vi "Teleop.vi"(10 "Match Info":T1={"Autonomous Elapsed Seconds"=0.0, "TeleOp Elapsed Seconds"=0.0, "Disabled Elapsed Seconds"=0.0, "Visited Autonomous"=FALSE, "Visited TeleOp"=FALSE, "Visited Disabled"=FALSE, "Autonomous Settings"={"Autonomous Style"=enum."Independent", "VI Refnum"=refnum}}, 11 "Call Context":T2) -> ()   [LabVIEW 2019]
doc: "This VI is called for each TeleOp packet received from the DS where the robot is not disabled. It is often used to read from the joysticks and update I/O or to update setpoints for timed control loops. It should complete and return within 20 milliseconds or it may miss DS packets."
uses:
  <vilib>/Rock Robotics/WPI/DriverStation/WPI_DriverStationDerivedRobotMode.ctl
  <vilib>/Rock Robotics/WPI/DriverStation/WPI_DriverStationMatch Info.ctl
  Robot Global Data.vi
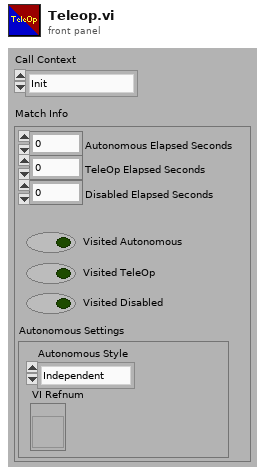
[diagram p1: front panel]
types:
  T1 = typedef "WPI_DriverStationMatch Info.ctl" = cluster{"Autonomous Elapsed Seconds":dbl, "TeleOp Elapsed Seconds":dbl, "Disabled Elapsed Seconds":dbl, "Visited Autonomous":bool, "Visited TeleOp":bool, "Visited Disabled":bool, "Autonomous Settings":cluster{"Autonomous Style":enum16{"Iterative", "Independent"}, "VI Refnum":refnum<vi>}}
  T2 = typedef "WPI_DriverStationDerivedRobotMode.ctl" = enum16{"Init", "Execute", "Stop"}
  T3 = typedef "WPI_JoystickDevRef.ctl" = cluster{"Device":T4}
  T4 = typedef "WPI_JoystickDeviceEnum.ctl" = enum16{"USB 0", "USB 1", "USB 2", "USB 3", "USB 4", "USB 5"}
  T5 = typedef "Color Sensor V3 DevRef.ctl" = cluster{"I2CDevRef":T6}
  T6 = typedef "WPI_I2CDevRef.ctl" = cluster{"DevStatus":errorcluster, "Device Address":u8, "Handle":i32, "I2C Bus":T7}
  T7 = typedef "i2c_bus.ctl" = enum16{"I2C On-Board", "I2C MXP", "Invalid"}
  T8 = typedef "WPI_EncoderDevRef.ctl" = cluster{"DevStatus":errorcluster, "EncoderIndex":T9, "CounterIndex":T10, "DistancePerCount":dbl, "Decoding Type":T11}
  T9 = typedef "FPGA_EncoderIdx.ctl" = enum8{"Enc 0", "Enc 1", "Enc 2", "Enc 3", "Enc 4", "Enc 5", "Enc 6", "Enc 7", "Invalid"}
  T10 = typedef "FPGA_CounterCtrSystemIndex.ctl" = enum8{"Ctr 0", "Ctr 1", "Ctr 2", "Ctr 3", "Ctr 4", "Ctr 5", "Ctr 6", "Ctr 7", "Invalid"}
  T11 = typedef "WPI_EncoderType.ctl" = enum16{"1x", "2x", "4x"}
  T12 = typedef "WPI_MotorControlDeviceRef.ctl" = cluster{"DeviceStatus":errorcluster, "Type":T13, "PWM":cluster{"PWM Channel":T14, "DeadBand":T15}, "CAN":cluster{"Device Number":u8, "SetOutput VI Ref":variant, "GetOutput VI Ref":variant, "Enable VI Ref":variant, "Disable VI Ref":variant, "Data":variant}, "Invert":bool, "DIO PWM":cluster{"PWM \"Enable\" Channel":T14, "DIOChannel":T16, "PWM Rate":dbl}}
  T13 = typedef "WPI_MotorControlType.ctl" = enum16{"PWM", "CAN", "DIO PWM"}
  T14 = typedef "FPGA_DIOPWMChannel.ctl" = enum8{"PWM 0", "PWM 1", "PWM 2", "PWM 3", "PWM 4", "PWM 5", "PWM 6", "PWM 7", "PWM 8", "PWM 9", "PWM MXP 0", "PWM MXP 1", "PWM MXP 2", "PWM MXP 3", "PWM MXP 4", "PWM MXP 5", "PWM MXP 6", "PWM MXP 7", "PWM MXP 8", "PWM MXP 9", "Invalid"}
  T15 = typedef "WPI_PWMDeadband.ctl" = cluster{"Name":string, "maxPositivePwm":i32, "minPositivePwm":i32, "centerPwm":i32, "maxNegativePwm":i32, "minNegativePwm":i32, "angularRange":u16}
  T16 = typedef "FPGA_DIOChannel.ctl" = enum8{"DIO 0", "DIO 1", "DIO 2", "DIO 3", "DIO 4", "DIO 5", "DIO 6", "DIO 7", "DIO 8", "DIO 9", "DIO MXP 0", "DIO MXP 1", "DIO MXP 2", "DIO MXP 3", "DIO MXP 4", "DIO MXP 5", "DIO MXP 6", "DIO MXP 7", "DIO MXP 8", "DIO MXP 9", "DIO MXP 10", "DIO MXP 11", "DIO MXP 12", "DIO MXP 13", "DIO MXP 14", "DIO MXP 15", "SPI Port CS1", "SPI Port CS2", "SPI Port CS3", "SPI Port MISO", "SPI Port MOSI", "Invalid"}
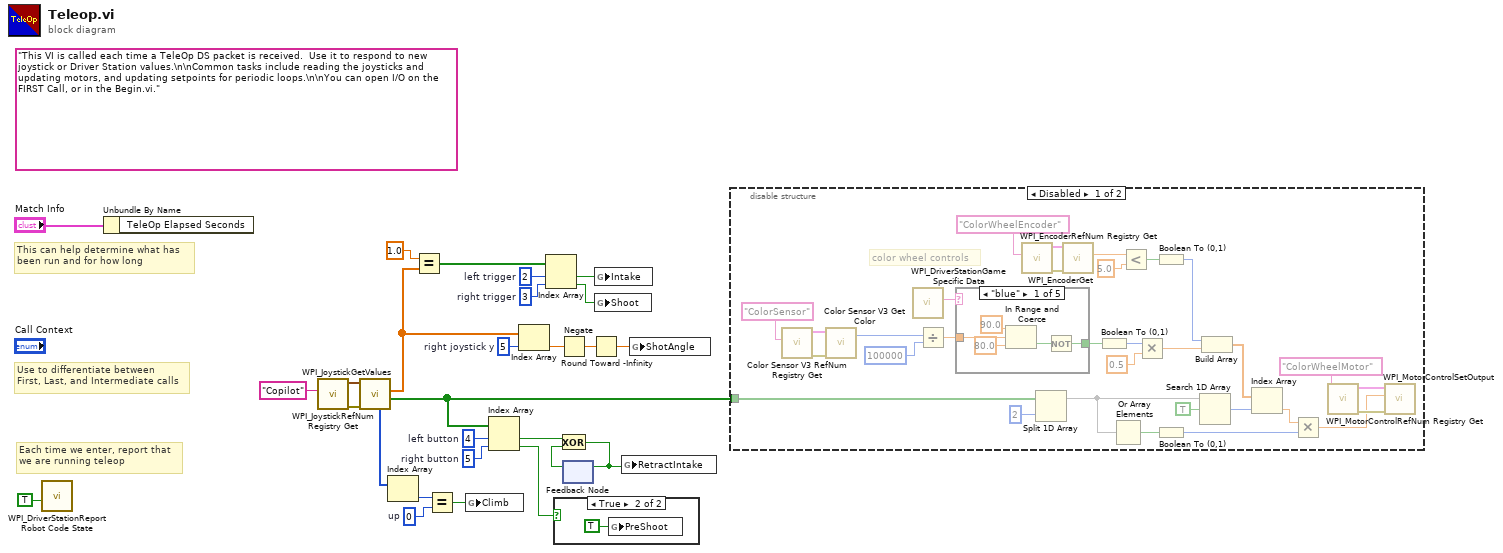
[diagram p0: block diagram]
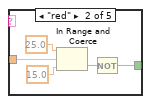
[diagram p3: hidden frame]
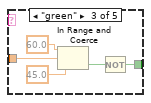
[diagram p4: hidden frame]
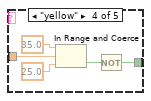
[diagram p5: hidden frame]
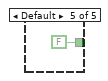
[diagram p6: hidden frame]
diagram:
  w11 = 5  # right joystick y
  w16 = i16 0  # up
  w22 = 5  # right button
  w23 = 4  # left button
  w24 = 3  # right trigger
  w25 = 2  # left trigger
  (unwired) "This VI is called each time a TeleOp DS packet is received.  Use it to respond to new joystick or Driver Station values.\n\nCommon tasks include reading the joysticks and updating motors, and updating setpoints for periodic loops.\n\nYou can open I/O on the FIRST Call, or in the Begin.vi."
  # "Each time we enter, report that\nwe are running teleop"
  # "Use to differentiate between\nFirst, Last, and Intermediate calls"
  # "This can help determine what has\nbeen run and for how long"
  n1 = call <vilib>:"WPI_DriverStationReport Robot Code State.vi"("TeleOp"=TRUE ("Autonomous")) -> ()  [unwired: 10 in, 1 out]
  n2 = Unbundle By Name("Match Info") -> ()  [unwired: 1 out]
  n3 = call <vilib>:"WPI_JoystickRefNum Registry Get.vi"("refnum name"="Copilot") -> ("error out"=w1:errorcluster, "JoystickDevRef"=w2:T3)  [unwired: 9 in]
  n4 = call <vilib>:"WPI_JoystickGetValues.vi"("error in (no error)"=w1, "JoystickDevRef"=w2) -> ("Buttons"=w13:bool[], "Axes"=w10:dbl[], "POVs"=w18:i16[])  [unwired: 5 in, 2 out]
  n5 = Index Array(array=w18) -> (element=w17:i16)  [unwired: 1 in]
  n6 = Equal?(x=1.0, y=w10) -> (x = y?=w21:bool[])
  n7 = Equal?(x=w17, y=w16) -> (x = y?=w15:bool)
  n8 = global write "Robot Global Data.vi" "Climb"(w15) -> ()
  n9 = Index Array(array=w13, index #1=w23, index #2=w22) -> (element #1=w5:bool, element #2=w7:bool)
  n10 = Index Array(array=w10, index=w11) -> (element=w9:dbl)
  n11 = Index Array(array=w21, index #1=w25, index #2=w24) -> (element #1=w19:bool, element #2=w14:bool)
  n12 = case shown="True" w7 {
    frame False {
    }
    frame True {
      n13 = global write "Robot Global Data.vi" "PreShoot"(TRUE ("PreShoot")) -> ()
    }
  }
  n14 = Negate(x=w9) -> (-x=w12:dbl)
  n15 = feedback #1() -> (w4:bool)  [unwired: 1 in]
  n16 = Exclusive Or(1:w4, 2:w5) -> (0:w6:bool)
  n17 = feedback-in #1(w6) -> ()
  n18 = Round Toward -Infinity(1:w12) -> (0:w8:dbl)
  n19 = global write "Robot Global Data.vi" "Intake"(w19) -> ()
  n20 = global write "Robot Global Data.vi" "Shoot"(w14) -> ()
  n21 = global write "Robot Global Data.vi" "RetractIntake"(w6) -> ()
  n22 = global write "Robot Global Data.vi" "ShotAngle"(w8) -> ()
  n23 = disable-structure shown="Disabled" {
    disable-tunnel: w13 -> [w30 _]
    frame Disabled {
      # "color wheel controls"
      n24 = call <vilib>:"Color Sensor V3 RefNum Registry Get.vi"("refnum name"="ColorSensor") -> ("error out"=w58:errorcluster, "ColorSensorDevRef"=w57:T5)  [unwired: 9 in]
      n25 = call <vilib>:"Color Sensor V3 Get Color.vi"("error in (no error)"=w58, "ColorSensorDevRef"=w57) -> ("Color"=w55:u32)  [unwired: 6 in, 3 out]
      n26 = call <vilib>:"WPI_DriverStationGame Specific Data.vi"() -> ("Game Specific Data"=w59:string)  [unwired: 11 in]
      n27 = Divide(x=w55, y=u32 100000) -> (x/y=w53:dbl)
      n28 = case shown="\"blue\"" w59 {
        tunnel: w53 -> [w64 w69 w74 w79 _]
        tunnel: [w60 w65 w70 w75 FALSE] -> w41
        frame "blue" {
          n29 = In Range and Coerce(upper limit=90.0, x=w64, lower limit=80.0) -> (In Range?=w61:bool)  [unwired: 1 out]
          n30 = Not(x=w61) -> (.not. x?=w60:bool)
        }
        frame "red" {
          n31 = In Range and Coerce(upper limit=25.0, x=w69, lower limit=15.0) -> (In Range?=w66:bool)  [unwired: 1 out]
          n32 = Not(x=w66) -> (.not. x?=w65:bool)
        }
        frame "green" {
          n33 = In Range and Coerce(upper limit=60.0, x=w74, lower limit=45.0) -> (In Range?=w71:bool)  [unwired: 1 out]
          n34 = Not(x=w71) -> (.not. x?=w70:bool)
        }
        frame "yellow" {
          n35 = In Range and Coerce(upper limit=35.0, x=w79, lower limit=25.0) -> (In Range?=w76:bool)  [unwired: 1 out]
          n36 = Not(x=w76) -> (.not. x?=w75:bool)
        }
        frame Default {
        }
      }
      n37 = call <vilib>:"WPI_EncoderRefNum Registry Get.vi"("refnum name"="ColorWheelEncoder") -> ("error out"=w39:errorcluster, "EncoderDevRef"=w40:T8)  [unwired: 9 in]
      n38 = Split 1D Array(array=w30, index=2) -> (first subarray=w29:bool[])  [unwired: 1 out]
      n39 = call <vilib>:"WPI_EncoderGet.vi"("error in (no error)"=w39, "EncoderDevRef"=w40) -> ("Distance"=w38:dbl)  [unwired: 4 in, 5 out]
      n40 = Boolean To (0,1)(Boolean=w41) -> (0, 1=w42:i16)
      n41 = Or Array Elements(Boolean array=w29) -> (logical OR=w47:bool)
      n42 = Less?(x=w38, y=5.0) -> (x < y?=w37:bool)
      n43 = Multiply(x=w42, y=0.5) -> (x*y=w48:dbl)
      n44 = Boolean To (0,1)(Boolean=w37) -> (0, 1=w34:i16)
      n45 = Boolean To (0,1)(Boolean=w47) -> (0, 1=w32:i16)
      n46 = Search 1D Array(1D array=w29, element=TRUE) -> (index of element=w45:i32)  [unwired: 1 in]
      n47 = Build Array(w34, w48) -> (w44:dbl[])
      n48 = Index Array(array=w44, index=w45) -> (element=w33:dbl)
      n49 = Multiply(x=w33, y=w32) -> (x*y=w43:dbl)
      n50 = call <vilib>:"WPI_MotorControlRefNum Registry Get.vi"("refnum name"="ColorWheelMotor") -> ("error out"=w50:errorcluster, "MotorControlDevRef"=w51:T12)  [unwired: 9 in]
      n51 = call <vilib>:"WPI_MotorControlSetOutput.vi"("error in (no error)"=w50, "Output"=w43, "MotorControlDevRef"=w51) -> ()  [unwired: 6 in, 3 out]
    }
    frame Enabled {
    }
  }
